vi "Init Analyze Objs from Report.vi"(8 "error in (no error)":errorcluster, 11 "refnum in":T1) -> (0 "error out":errorcluster, 1 "All Objects":refnum<class "Analyze BaseClass.lvclass">[](array[class]), 2 "Selected Objs":refnum<class "Analyze BaseClass.lvclass">[](array[class]), 3 "refnum out":T1)   [LabVIEW 2020, in "POLARIS IMAQ Display.xctl"]
uses:
  POLARIS IMAQ Display.xctl
  Analyze Classes/Analyze BaseClass/Analyze BaseClass.lvclass
  <vilib>/Utility/config.llb/Config Data RefNum.ctl
  Analyze Classes/Analyze.lvlib
  <vilib>/Utility/config.llb/NI_LVConfig.lvlib
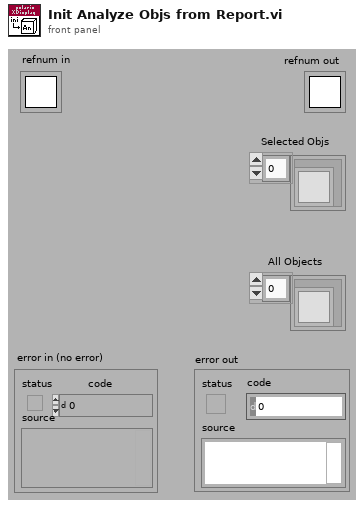
[diagram p1: front panel]
types:
  T1 = typedef "NI_LVConfig.lvlib/Config Data RefNum.ctl" = refnum<k1>
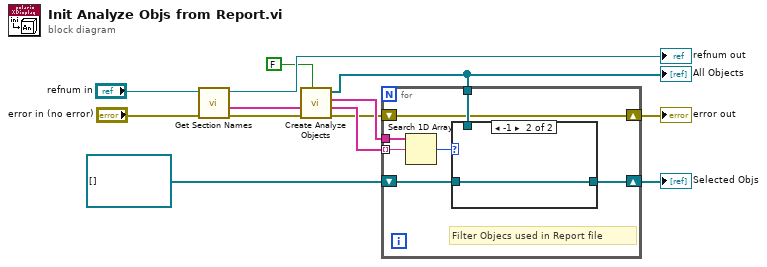
[diagram p0: block diagram]
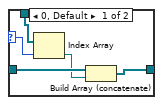
[diagram p2: hidden frame]
diagram:
  n1 = call <vilib>:"Get Section Names.vi"("error in (no error)"="error in (no error)", "refnum"="refnum in") -> ("error out"=w5:errorcluster, "section names"=w10:string[], "refnum out"=→"refnum out":T1)  [unwired: 7 in]
  n2 = call "Create Analyze Objects.vi"("Reload"=FALSE, "error in (no error)"=w5) -> ("error out"=w4:errorcluster, "Short Name"=w9:string[], "Objects"=w7:refnum<class "Analyze BaseClass.lvclass">[])  [unwired: 7 in]
  "All Objects" <- w7
  n3 = for {
    tunnel: w10 -> [w14] mode=indexing
    shift-right: [w13] -> w2
    shift-left: w4 -> [w13]
    tunnel: w9 -> [w15]
    shift-right: [w17] -> w3
    shift-left: refnum<class "Analyze BaseClass.lvclass">[] [] ("Selected Objs") -> [w18]
    tunnel: w7 -> [w16]
    # "Filter Objecs used in Report file"
    n4 = Search 1D Array(1D array=w15, element=w14) -> (index of element=w19:i32)  [unwired: 1 in]
    n5 = case shown="-1" w19 {
      selector: w19 -> [w23 _]
      tunnel: w18 -> [w24 w25]
      tunnel: [w20 w25] -> w17
      tunnel: w16 -> [w22 _]
      frame 0, Default {
        n6 = Index Array(array=w22, index=w23) -> (element=w21:refnum<class "Analyze BaseClass.lvclass">)
        n7 = Build Array (concatenate)(w24, w21) -> (w20:refnum<class "Analyze BaseClass.lvclass">[])
      }
      frame -1 {
      }
    }
  }
  "error out" <- w2
  "Selected Objs" <- w3
